vi "Spartan Builder - Build Help Files.vi"(8 "error in":errorcluster) -> (0 "error out":errorcluster)   [LabVIEW 2011]
doc: "Use this VI Template to create a custom Pre-/Post-Build VI."
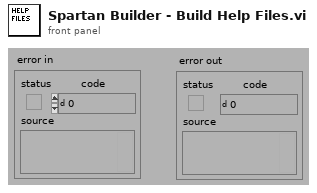
[diagram p1: front panel]
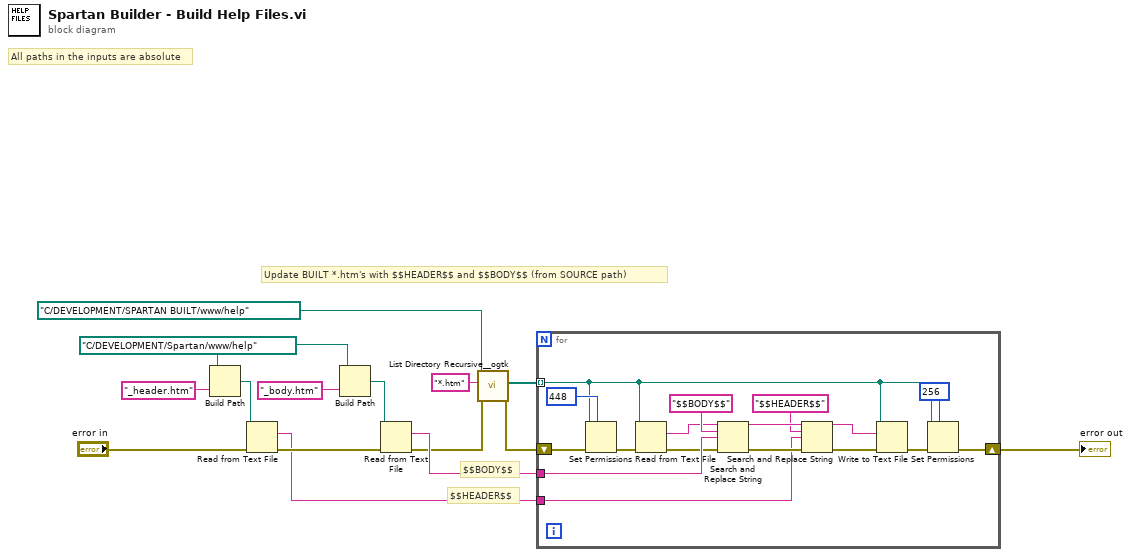
[diagram p0: block diagram]
diagram:
  w2 = path "C:/DEVELOPMENT/Spartan/www/help" ("Build Parameters v0.0.Source Root")
  # "Update BUILT *.htm's with $$HEADER$$ and $$BODY$$ (from SOURCE path)"
  # "$$BODY$$"
  # "$$HEADER$$"
  # "All paths in the inputs are absolute"
  n1 = Build Path(base path=w2, name or relative path="_header.htm") -> (appended path=w12:path)
  n2 = Read from Text File(file (use dialog)=w12, error in="error in") -> (text=w8:string, error out=w13:errorcluster)  [unwired: 4 out]
  n3 = Build Path(base path=w2, name or relative path="_body.htm") -> (appended path=w9:path)
  n4 = Read from Text File(file (use dialog)=w9, error in=w13) -> (text=w7:string, error out=w6:errorcluster)  [unwired: 4 out]
  n5 = call "List Directory Recursive__ogtk.vi"("error in (no error)"=w6, "pattern"="*.htm", "Path"=path "C:/DEVELOPMENT/SPARTAN BUILT/www/help" ("Build Parameters v0.0.Source Root")) -> ("error out"=w5:errorcluster, "file paths"=w4:path[])  [unwired: 2 in, 5 out]
  n6 = for {
    shift-right: [w18] -> w15
    shift-left: w5 -> [w22]
    tunnel: w8 -> [w26]
    tunnel: w7 -> [w29]
    tunnel: w4 -> [w16] mode=indexing
    n7 = Set Permissions(7:i16 448 ("permissions"), 8:w22, 11:w16) -> (0:w21:errorcluster)  [unwired: 3 out]
    n8 = Read from Text File(file (use dialog)=w16, error in=w21) -> (text=w31:string, error out=w28:errorcluster)  [unwired: 4 out]
    n9 = Search and Replace String(input string=w31, search string="$$BODY$$", replace string=w29, error in=w28) -> (result string=w30:string, error out=w27:errorcluster)  [unwired: 6 out]
    n10 = Search and Replace String(input string=w30, search string="$$HEADER$$", replace string=w26, error in=w27) -> (result string=w23:string, error out=w24:errorcluster)  [unwired: 6 out]
    n11 = Write to Text File(file (use dialog)=w16, text=w23, error in=w24) -> (error out=w19:errorcluster)  [unwired: 3 out]
    n12 = Set Permissions(7:i16 256 ("permissions"), 8:w19, 11:w16) -> (0:w18:errorcluster)  [unwired: 3 out]
  }
  "error out" <- w15
